vi "Read Message Priority (Normal).vi"(8 "error in (no error)":errorcluster, 11 "Self-addressed Msg in":refnum<class "Self-addressed Msg.lvclass">) -> (0 "error out":errorcluster, 2 "Message Priority":T1=enum."Normal", 3 "Self-addressed Msg out":refnum<class "Self-addressed Msg.lvclass">)   [LabVIEW 2019, in "Self-addressed Msg.lvclass"]
uses:
  Self-addressed Msg.lvclass
  <vilib>/ActorFramework/Message Enqueuer/Message Priority.ctl
  Self-addressed Msg.lvclass/Self-addressed Msg.ctl
  <vilib>/ActorFramework/Message Enqueuer/Message Enqueuer.lvclass
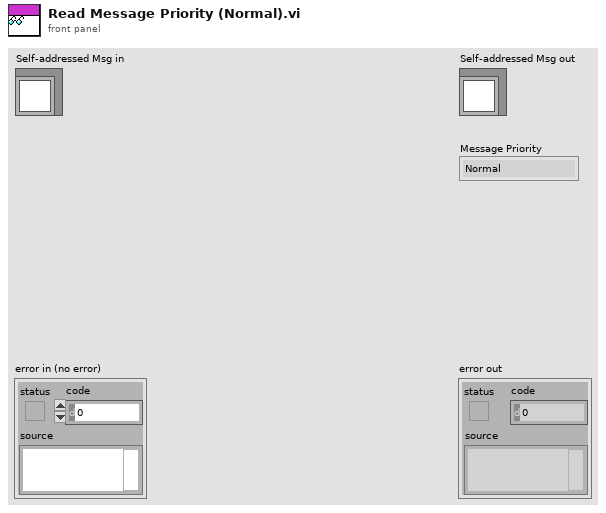
[diagram p1: front panel]
types:
  T1 = typedef "Actor Framework.lvlib/Message Enqueuer.lvclass/Message Priority.ctl" = enum16{"Low", "Normal", "High"}
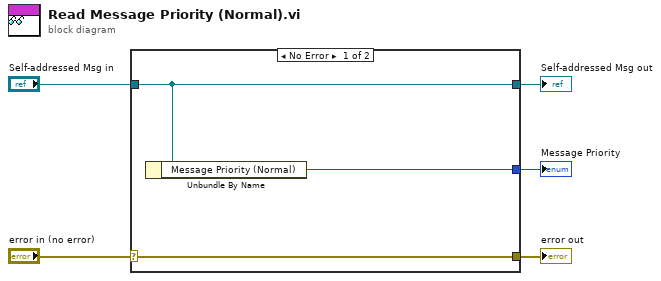
[diagram p0: block diagram]
diagram:
  n1 = case shown="No Error" "error in (no error)" {
    selector: "error in (no error)" -> [w8 w9]
    tunnel: [w8 w9] -> w4
    tunnel: [w7 w10] -> w2
    tunnel: "Self-addressed Msg in" -> [w7 w10]
    tunnel: [w6 _] -> w1
    frame No Error {
      n2 = Unbundle By Name(w7) -> ("Message Priority (Normal)"=w6:T1)
    }
    frame Error {
    }
  }
  "error out" <- w4
  "Self-addressed Msg out" <- w2
  "Message Priority" <- w1
